vi "ComSelect.vi"(2 "error in":errorcluster caption="错误输入（无错误）", 3 "CAN通路":T1(ring)) -> (0 "error out":errorcluster caption="错误输出", 1 "COM1":refnum<visa-resource-name>)   [LabVIEW 2013]
uses:
  Global.vi
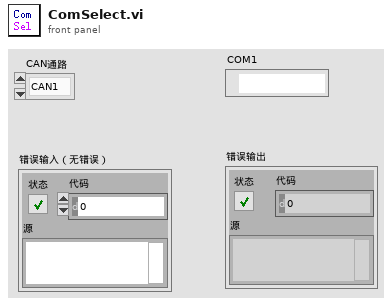
[diagram p1: front panel]
types:
  T1 = enum16{"CAN1", "CAN2", "CAN3", "CAN4", "CAN5", "CAN6", "CAN7", "CAN8"}
  T2 = cluster{"COM1":refnum<visa-resource-name>, "COM2":refnum<visa-resource-name>, "COM3":refnum<visa-resource-name>, "COM4":refnum<visa-resource-name>, "COM5":refnum<visa-resource-name>, "COM6":refnum<visa-resource-name>, "COM7":refnum<visa-resource-name>, "COM8":refnum<visa-resource-name>}
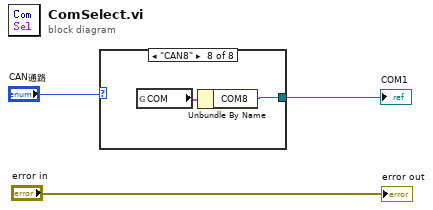
[diagram p0: block diagram]
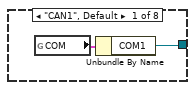
[diagram p2: hidden frame]
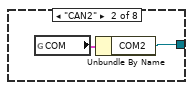
[diagram p3: hidden frame]
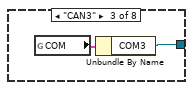
[diagram p4: hidden frame]
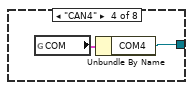
[diagram p5: hidden frame]
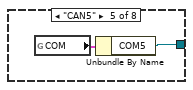
[diagram p6: hidden frame]
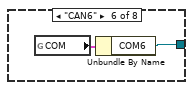
[diagram p7: hidden frame]
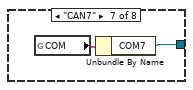
[diagram p8: hidden frame]
diagram:
  n1 = case shown="\"CAN8\"" "CAN通路" {
    tunnel: [w4 w6 w8 w10 w12 w14 w16 w18] -> w2
    frame "CAN1", Default {
      n2 = global read "Global.vi" "COM"() -> (w5:T2)
      n3 = Unbundle By Name(w5) -> ("COM1"=w4:refnum<visa-resource-name>)
    }
    frame "CAN2" {
      n4 = global read "Global.vi" "COM"() -> (w7:T2)
      n5 = Unbundle By Name(w7) -> ("COM2"=w6:refnum<visa-resource-name>)
    }
    frame "CAN3" {
      n6 = global read "Global.vi" "COM"() -> (w9:T2)
      n7 = Unbundle By Name(w9) -> ("COM3"=w8:refnum<visa-resource-name>)
    }
    frame "CAN4" {
      n8 = global read "Global.vi" "COM"() -> (w11:T2)
      n9 = Unbundle By Name(w11) -> ("COM4"=w10:refnum<visa-resource-name>)
    }
    frame "CAN5" {
      n10 = global read "Global.vi" "COM"() -> (w13:T2)
      n11 = Unbundle By Name(w13) -> ("COM5"=w12:refnum<visa-resource-name>)
    }
    frame "CAN6" {
      n12 = global read "Global.vi" "COM"() -> (w15:T2)
      n13 = Unbundle By Name(w15) -> ("COM6"=w14:refnum<visa-resource-name>)
    }
    frame "CAN7" {
      n14 = global read "Global.vi" "COM"() -> (w17:T2)
      n15 = Unbundle By Name(w17) -> ("COM7"=w16:refnum<visa-resource-name>)
    }
    frame "CAN8" {
      n16 = global read "Global.vi" "COM"() -> (w19:T2)
      n17 = Unbundle By Name(w19) -> ("COM8"=w18:refnum<visa-resource-name>)
    }
  }
  "COM1" <- w2
  "error out" <- "error in"
